vi "hostDataLogger.vi"() -> ()   [LabVIEW 2018]
uses:
  <vilib>/Utility/file.llb/Write Delimited Spreadsheet (DBL).vi
panel:
  out "Modified Value = Ax+B":dbl
  in  "B":dbl=1.0
  in  "A":dbl=1.0 format="%#_13g"
  in  "Stop cRIO":bool
  in  "Sampling Period (ms)":u32=100
  in  "Save to File":bool
  out "Current Value":dbl
  out "Live Data":dbl(graph)
  out "Recorded Data":string[][](table)
  in  "Stop Host":bool
  in  "Flush Data":bool
  in  "Record Data":bool
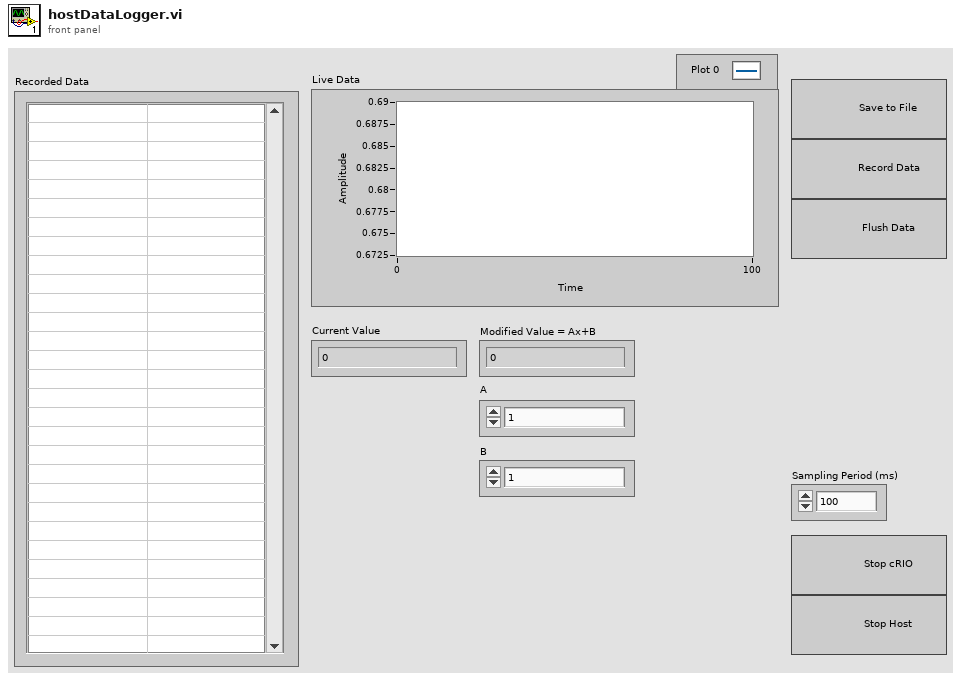
[diagram p1: front panel]
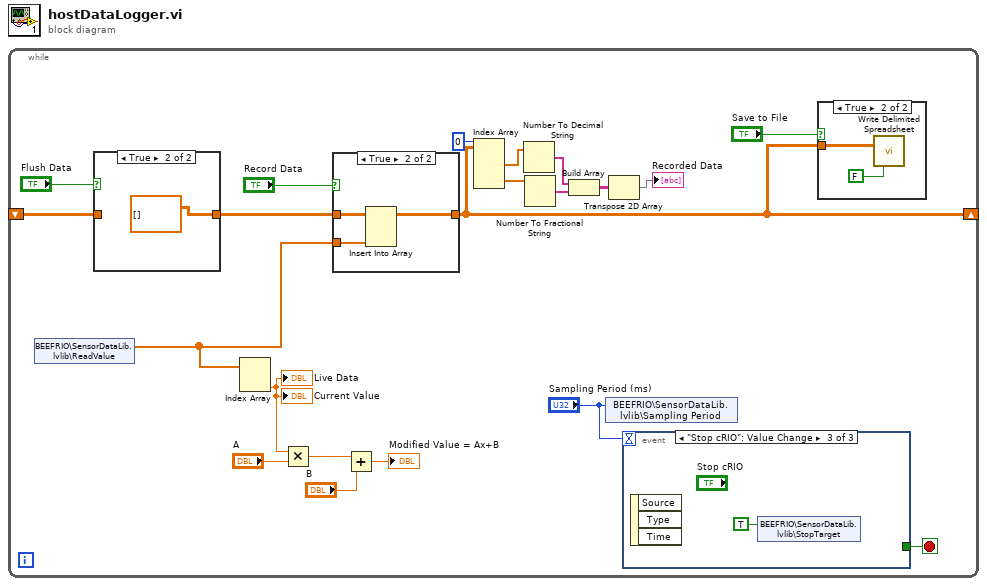
[diagram p0: block diagram]
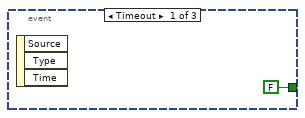
[diagram p5: hidden frame]
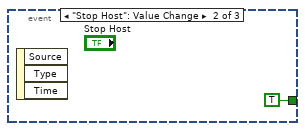
[diagram p6: hidden frame]
diagram:
  n1 = while {
    shift-right: [w4] -> _
    shift-left: _ -> [w18]
    stop <- w21 stop-if-true
    n2 = shared-variable "BEEFRIO\\SensorDataLib.lvlib\\ReadValue"() -> (w16:dbl[])  [unwired: 1 in, 1 out]
    n3 = case shown="True" "Flush Data" {
      tunnel: w18 -> [w24 _]
      tunnel: [w24 dbl[][] []] -> w17
      frame False {
      }
      frame True {
      }
    }
    n4 = Index Array(array=w16) -> (element #2=w1:dbl)  [unwired: 2 in, 1 out]
    "Live Data" <- w1
    "Current Value" <- w1
    n5 = Multiply(x=w1, y="A") -> (x*y=w7:dbl)
    n6 = case shown="True" "Record Data" {
      tunnel: w16 -> [_ w27]
      tunnel: [w26 w29] -> w4
      tunnel: w17 -> [w26 w28]
      frame False {
      }
      frame True {
        n7 = Insert Into Array(array=w28, new element=w27) -> (w29:dbl[][])  [unwired: 2 in]
      }
    }
    n8 = Add(x=w7, y="B") -> (x+y=→"Modified Value = Ax+B":dbl)
    n9 = Index Array(array=w4, index (col) #1=0 ("disabled index (col)")) -> (element #1=w14:dbl[], element #2=w2:dbl[])  [unwired: 3 in]
    n10 = Number To Decimal String(number=w14) -> (decimal integer string=w13:string[])  [unwired: 1 in]
    n11 = Number To Fractional String(number=w2) -> (F-format string=w12:string[])  [unwired: 3 in]
    n12 = Build Array(w13, w12) -> (w11:string[][])
    n13 = shared-variable "BEEFRIO\\SensorDataLib.lvlib\\Sampling Period"("Sampling Period (ms)") -> ()  [unwired: 1 in, 1 out]
    n14 = Transpose 2D Array(2D array=w11) -> (transposed array=→"Recorded Data":string[][])
    n15 = event shown="[2] \"Stop cRIO\": Value Change" {
      selector: _ -> [_ _ _]
      dyn-events: _ -> [_ _ _]
      timeout: "Sampling Period (ms)" -> [_ _ _]
      tunnel: [FALSE TRUE _] -> w21
      event Timeout {
        n16 = event-data() -> ()  [unwired: 1 in, 3 out]
      }
      event "Stop Host": Value Change {
        n17 = event-data() -> ()  [unwired: 1 in, 3 out]
      }
      event "Stop cRIO": Value Change {
        n18 = event-data() -> ()  [unwired: 1 in, 3 out]
        n19 = shared-variable "BEEFRIO\\SensorDataLib.lvlib\\StopTarget"(TRUE ("StopTarget")) -> ()  [unwired: 1 in, 1 out]
      }
    }
    n20 = case shown="True" "Save to File" {
      tunnel: w4 -> [_ w23]
      frame False {
      }
      frame True {
        n21 = call-poly <vilib>:"Write Delimited Spreadsheet.vi"("2D data"=w23, "transpose? (no:F)"=FALSE) -> ()  [unwired: 12 in, 2 out]
      }
    }
  }
